vi "Failure Message.vi"() -> ()   [LabVIEW 2017, in "Transparent Assertions.Tests.lvlib" / "Assert Error.lvlib"]
uses:
  Assert Error.lvlib
  src/Transparent Assertions/Transparent Assertions.lvlib
panel:
  out "error out":errorcluster
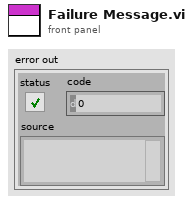
[diagram p1: front panel]
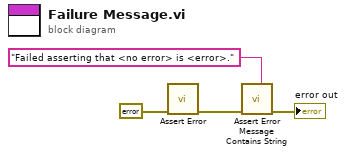
[diagram p0: block diagram]
diagram:
  n1 = call "Assert Error.vi"("error in (no error)"=errorcluster {"status"=FALSE, "code"=0, "source"=""}) -> ("error out"=w3:errorcluster)  [unwired: 10 in]
  n2 = call "Assert Error Message Contains String.vi"("Expected"="Failed asserting that <no error> is <error>.", "error in (no error)"=w3) -> ("error out"=→"error out":errorcluster)  [unwired: 9 in]
